vi "Lichtgitter_Referenzen_aufnehmen.vi"(8 "Fehler in":errorcluster, 11 "Cluster in":T1={"Initialisierung"={"Online?"=FALSE, "Grundpfad"=path "", "Kamera Oben"="", "IP-Adresse Flüssiglinse"="", "Flüssiglinse"=refnum, "Kamera Unten"="", "IP-Adresse SPS"="", "SPS-Verbindung"={"TCP Connection Ref"=refnum, "IP address"="", "timeout ms"=5000, "Connected?"=FALSE, "PLC Type"=enum."S7 1200", "Rack S7 400"=0, "Slot S7 400"=0, "PDU Size"=0, "connection semaphore"=refnum}, "IP-Adresse Lichtgitter"="", "Lichtgitter"=refnum, "Skalierungsfaktor"=0.0, "Bilder Oben"=[], "Bild Unten"=refnum, "Bild Ausschnitt Unten"=refnum}, "Einstellungen"={"Gesamtablauf gestartet"=FALSE, "i. O. Bilder speichern"=FALSE, "Bildspeicherung Offline"=FALSE, "Ausgewähltes Offline-Datum"="", "Ausgewähltes Offline-Teil"="", "Speicherpfad Bilder"=path ""}, "Artikeldaten"={"Artikelnummer"="", "Fertigungsauftrag"="", "Muster ISO"=refnum, "Belichtungszeit Referenzmarken"=0.0, "Fokus Referenzmarken"=0.0, "Belichtungszeit ISO"=0.0, "Fokus ISO"=0.0, "Belichtungszeit Unten"=0.0, "Kontaktanzahl"=0, "Aktueller Kontakt"=0, "Kontaktposition"={"x"=0.0, "y"=0.0}, "ISO-Muster nicht vorhanden"=FALSE, "Winkel ISO"=0.0, "Mittelpunkt ISO"={"x"=0.0, "y"=0.0}}, "Werte Kamera Oben"={"Koordinatensystem"={"Punkt x-Achse"={"X"=0.0, "Y"=0.0}, "Ursprung"={"X"=0.0, "Y"=0.0}, "Punkt y-Achse"={"X"=0.0, "Y"=0.0}}, "Position Kontakt"={"x"=0.0, "y"=0.0}, "Durchmesser Loch"=0.0, "Winkel Kontakt"=0.0, "Position Kontakt umgerechnet"={"x"=0.0, "y"=0.0}}, "Werte Kamera Unten"={"Prüfung Unten n. i. O."=FALSE}, "Werte Lichtgitter"={"Messwerte Referenzmarken"=[], "Mittelpunkt Referenzmarken"={"x"=0.0, "y"=0.0}, "Messwerte Kontakt"=[], "Offset"={"x"=0.0, "y"=0.0}}, "Rückmeldungen"={"Koordinaten ermittelt"=FALSE, "Vermessung Lichtgitter fertig"=FALSE, "Nachkontrolle Kamera Unten fertig"=FALSE}, "Fehler"={"Referenzen nicht gefunden"=FALSE, "Kontakt nicht gefunden"=FALSE, "Referenzen nicht in Lichtgitter"=FALSE, "Kontakt zu groß"=FALSE, "Kontakt zu klein"=FALSE}, "Statistik"={"Statistiken"=[]}, "Timer"={"Timer Start Position"=0, "Timer Start Lichtgitter"=0, "Timer Start Kamera Unten"=0}}) -> (0 "Fehler out":errorcluster, 3 "Cluster out":T1={"Initialisierung"={"Online?"=FALSE, "Grundpfad"=path "", "Kamera Oben"="", "IP-Adresse Flüssiglinse"="", "Flüssiglinse"=refnum, "Kamera Unten"="", "IP-Adresse SPS"="", "SPS-Verbindung"={"TCP Connection Ref"=refnum, "IP address"="", "timeout ms"=5000, "Connected?"=FALSE, "PLC Type"=enum."S7 1200", "Rack S7 400"=0, "Slot S7 400"=0, "PDU Size"=0, "connection semaphore"=refnum}, "IP-Adresse Lichtgitter"="", "Lichtgitter"=refnum, "Skalierungsfaktor"=0.0, "Bilder Oben"=[], "Bild Unten"=refnum, "Bild Ausschnitt Unten"=refnum}, "Einstellungen"={"Gesamtablauf gestartet"=FALSE, "i. O. Bilder speichern"=FALSE, "Bildspeicherung Offline"=FALSE, "Ausgewähltes Offline-Datum"="", "Ausgewähltes Offline-Teil"="", "Speicherpfad Bilder"=path ""}, "Artikeldaten"={"Artikelnummer"="", "Fertigungsauftrag"="", "Muster ISO"=refnum, "Belichtungszeit Referenzmarken"=0.0, "Fokus Referenzmarken"=0.0, "Belichtungszeit ISO"=0.0, "Fokus ISO"=0.0, "Belichtungszeit Unten"=0.0, "Kontaktanzahl"=0, "Aktueller Kontakt"=0, "Kontaktposition"={"x"=0.0, "y"=0.0}, "ISO-Muster nicht vorhanden"=FALSE, "Winkel ISO"=0.0, "Mittelpunkt ISO"={"x"=0.0, "y"=0.0}}, "Werte Kamera Oben"={"Koordinatensystem"={"Punkt x-Achse"={"X"=0.0, "Y"=0.0}, "Ursprung"={"X"=0.0, "Y"=0.0}, "Punkt y-Achse"={"X"=0.0, "Y"=0.0}}, "Position Kontakt"={"x"=0.0, "y"=0.0}, "Durchmesser Loch"=0.0, "Winkel Kontakt"=0.0, "Position Kontakt umgerechnet"={"x"=0.0, "y"=0.0}}, "Werte Kamera Unten"={"Prüfung Unten n. i. O."=FALSE}, "Werte Lichtgitter"={"Messwerte Referenzmarken"=[], "Mittelpunkt Referenzmarken"={"x"=0.0, "y"=0.0}, "Messwerte Kontakt"=[], "Offset"={"x"=0.0, "y"=0.0}}, "Rückmeldungen"={"Koordinaten ermittelt"=FALSE, "Vermessung Lichtgitter fertig"=FALSE, "Nachkontrolle Kamera Unten fertig"=FALSE}, "Fehler"={"Referenzen nicht gefunden"=FALSE, "Kontakt nicht gefunden"=FALSE, "Referenzen nicht in Lichtgitter"=FALSE, "Kontakt zu groß"=FALSE, "Kontakt zu klein"=FALSE}, "Statistik"={"Statistiken"=[]}, "Timer"={"Timer Start Position"=0, "Timer Start Lichtgitter"=0, "Timer Start Kamera Unten"=0}})   [LabVIEW 2024]
uses:
  Typdefinitionen/Cluster.ctl
  <vilib>/userDefined/High Color/IMAQdx.ctl
  <vilib>/DATA AHEAD/SP7/typedefs/S7 Connection.ctl
  <vilib>/DATA AHEAD/SP7/typedefs/PLC Type.ctl
  <vilib>/vision/Image Controls.llb/IMAQ Image.ctl
  Typdefinitionen/Koordinatensystem.ctl
  Typdefinitionen/Statistik.ctl
  <vilib>/Utility/file.llb/Read Delimited Spreadsheet (DBL).vi
  <vilib>/DATA AHEAD/SP7/SP7.lvlib
panel:
  out "Zeit":u32
  out "Anzahl Kanten":i32[](array[numeric])
  out "Lese- und Schreibestrings":string
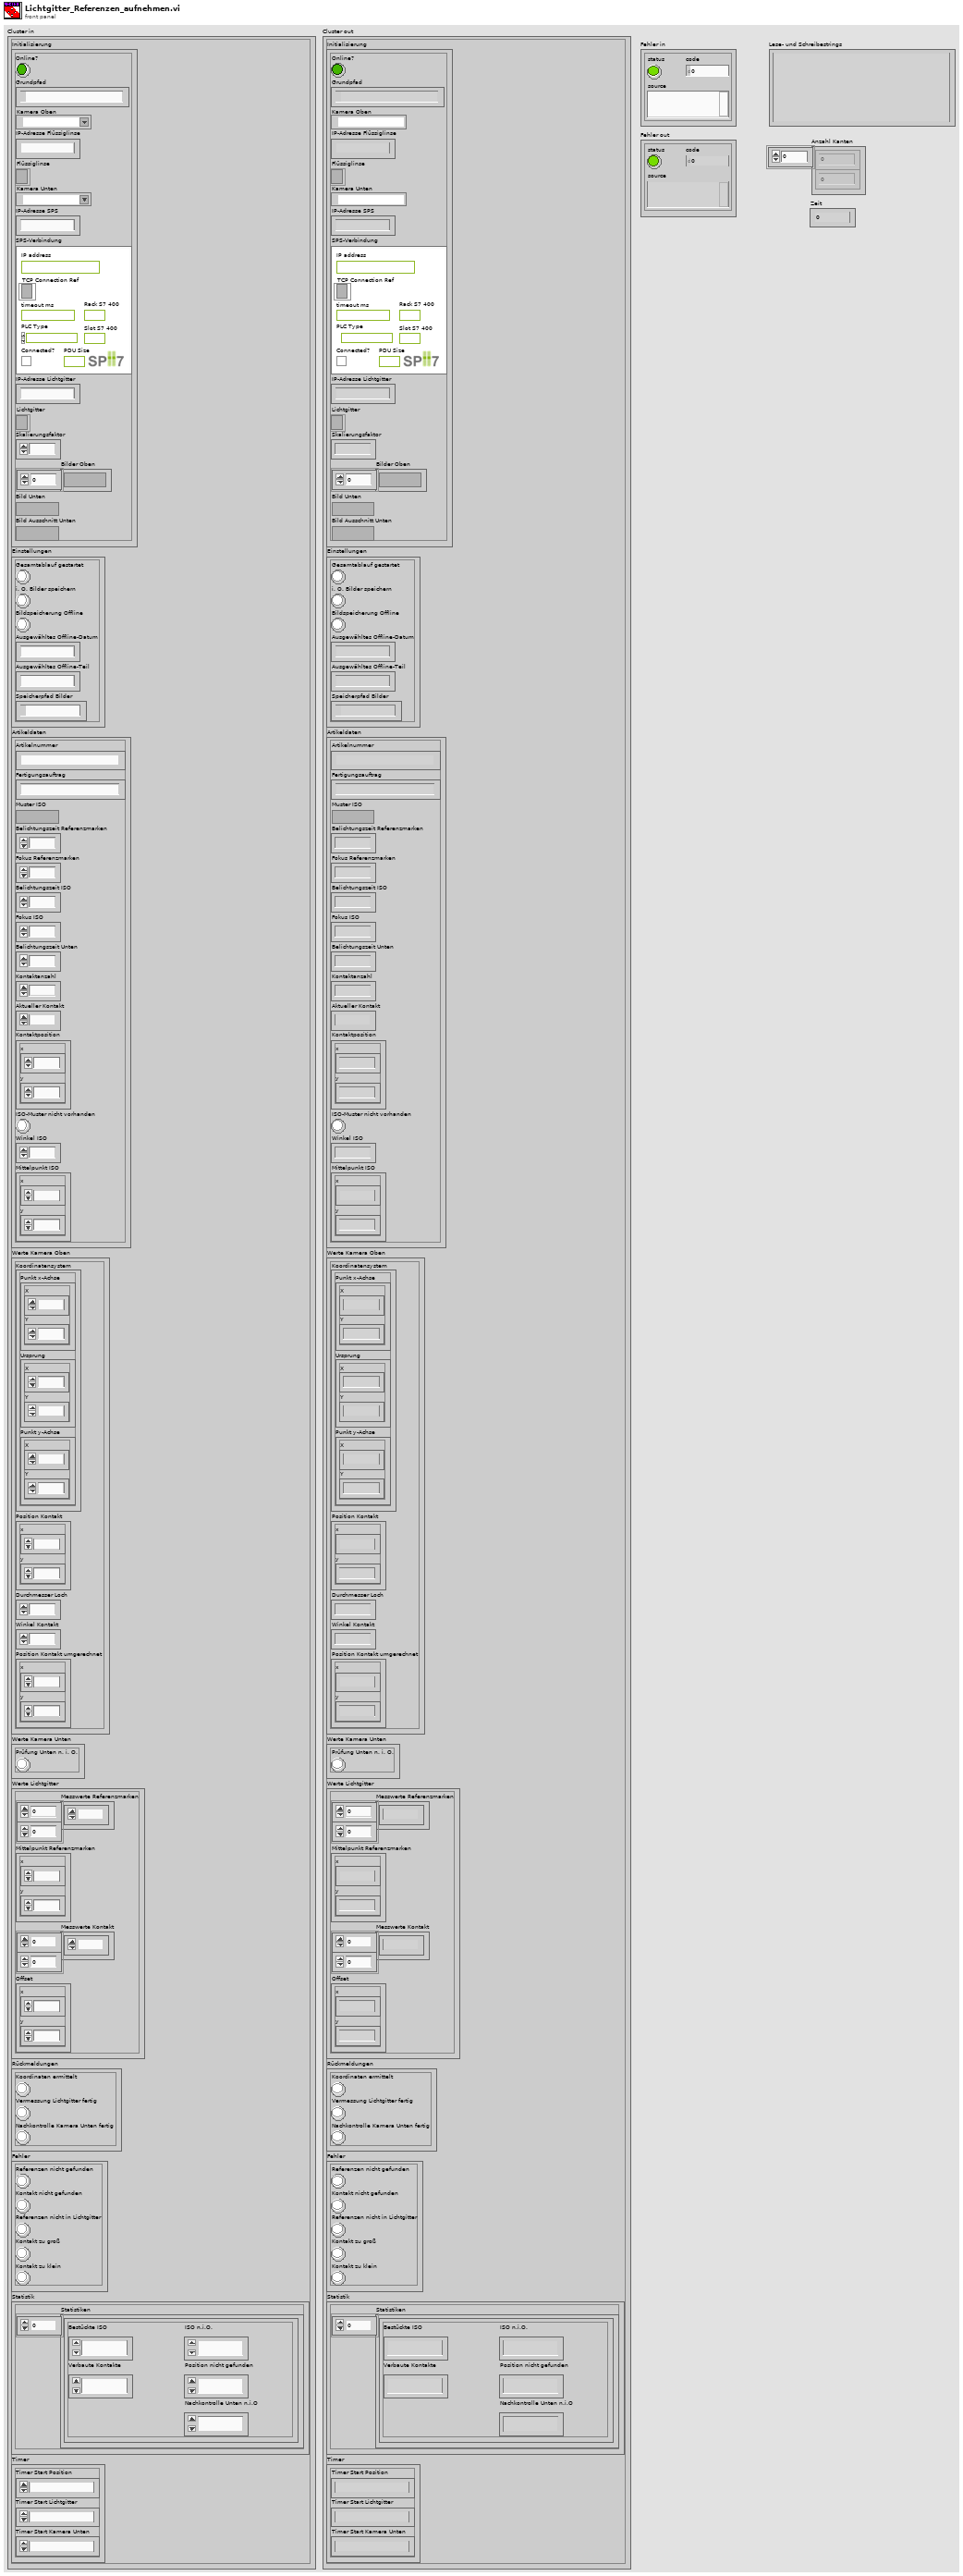
[diagram p1: front panel]
types:
  T1 = typedef "Cluster.ctl" = cluster{"Initialisierung":cluster{"Online?":bool, "Grundpfad":path, "Kamera Oben":T2, "IP-Adresse Flüssiglinse":string, "Flüssiglinse":refnum<k5>, "Kamera Unten":T2, "IP-Adresse SPS":string, "SPS-Verbindung":T3, "IP-Adresse Lichtgitter":string, "Lichtgitter":refnum<k5>, "Skalierungsfaktor":dbl, "Bilder Oben":T6[], "Bild Unten":T6, "Bild Ausschnitt Unten":T6}, "Einstellungen":cluster{"Gesamtablauf gestartet":bool, "i. O. Bilder speichern":bool, "Bildspeicherung Offline":bool, "Ausgewähltes Offline-Datum":string, "Ausgewähltes Offline-Teil":string, "Speicherpfad Bilder":path}, "Artikeldaten":cluster{"Artikelnummer":string, "Fertigungsauftrag":string, "Muster ISO":T6, "Belichtungszeit Referenzmarken":dbl, "Fokus Referenzmarken":dbl, "Belichtungszeit ISO":dbl, "Fokus ISO":dbl, "Belichtungszeit Unten":dbl, "Kontaktanzahl":u32, "Aktueller Kontakt":i16, "Kontaktposition":cluster{"x":sgl, "y":sgl}, "ISO-Muster nicht vorhanden":bool, "Winkel ISO":sgl, "Mittelpunkt ISO":cluster{"x":dbl, "y":dbl}}, "Werte Kamera Oben":cluster{"Koordinatensystem":T7, "Position Kontakt":cluster{"x":dbl, "y":dbl}, "Durchmesser Loch":dbl, "Winkel Kontakt":dbl, "Position Kontakt umgerechnet":cluster{"x":dbl, "y":dbl}}, "Werte Kamera Unten":cluster{"Prüfung Unten n. i. O.":bool}, "Werte Lichtgitter":cluster{"Messwerte Referenzmarken":dbl[][], "Mittelpunkt Referenzmarken":cluster{"x":dbl, "y":dbl}, "Messwerte Kontakt":dbl[][], "Offset":cluster{"x":dbl, "y":dbl}}, "Rückmeldungen":cluster{"Koordinaten ermittelt":bool, "Vermessung Lichtgitter fertig":bool, "Nachkontrolle Kamera Unten fertig":bool}, "Fehler":cluster{"Referenzen nicht gefunden":bool, "Kontakt nicht gefunden":bool, "Referenzen nicht in Lichtgitter":bool, "Kontakt zu groß":bool, "Kontakt zu klein":bool}, "Statistik":cluster{"Statistiken":T8[]}, "Timer":cluster{"Timer Start Position":u32, "Timer Start Lichtgitter":u32, "Timer Start Kamera Unten":u32}}
  T2 = typedef "IMAQdx.ctl" = refnum<k21>
  T3 = typedef "SP7.lvlib/S7 Connection.ctl" = cluster{"TCP Connection Ref":refnum<k5>, "IP address":string, "timeout ms":i32, "Connected?":bool, "PLC Type":T4, "Rack S7 400":u8, "Slot S7 400":u8, "PDU Size":u16, "connection semaphore":T5}
  T4 = typedef "SP7.lvlib/PLC Type.ctl" = enum16{"S7 200", "S7 300/400", "S7 1200", "S7 1500", "LOGO!8"}
  T5 = typedef "Semaphore RefNum" = refnum<k1>
  T6 = typedef "IMAQ Image.ctl" = refnum<image>
  T7 = typedef "Koordinatensystem.ctl" = cluster{"Punkt x-Achse":cluster{"X":sgl, "Y":sgl}, "Ursprung":cluster{"X":sgl, "Y":sgl}, "Punkt y-Achse":cluster{"X":sgl, "Y":sgl}}
  T8 = typedef "Statistik.ctl" = cluster{"Bestückte ISO":u32, "Verbaute Kontakte":u32, "ISO n.i.O.":u32, "Nachkontrolle Unten n.i.O":u32, "Position nicht gefunden":u32}
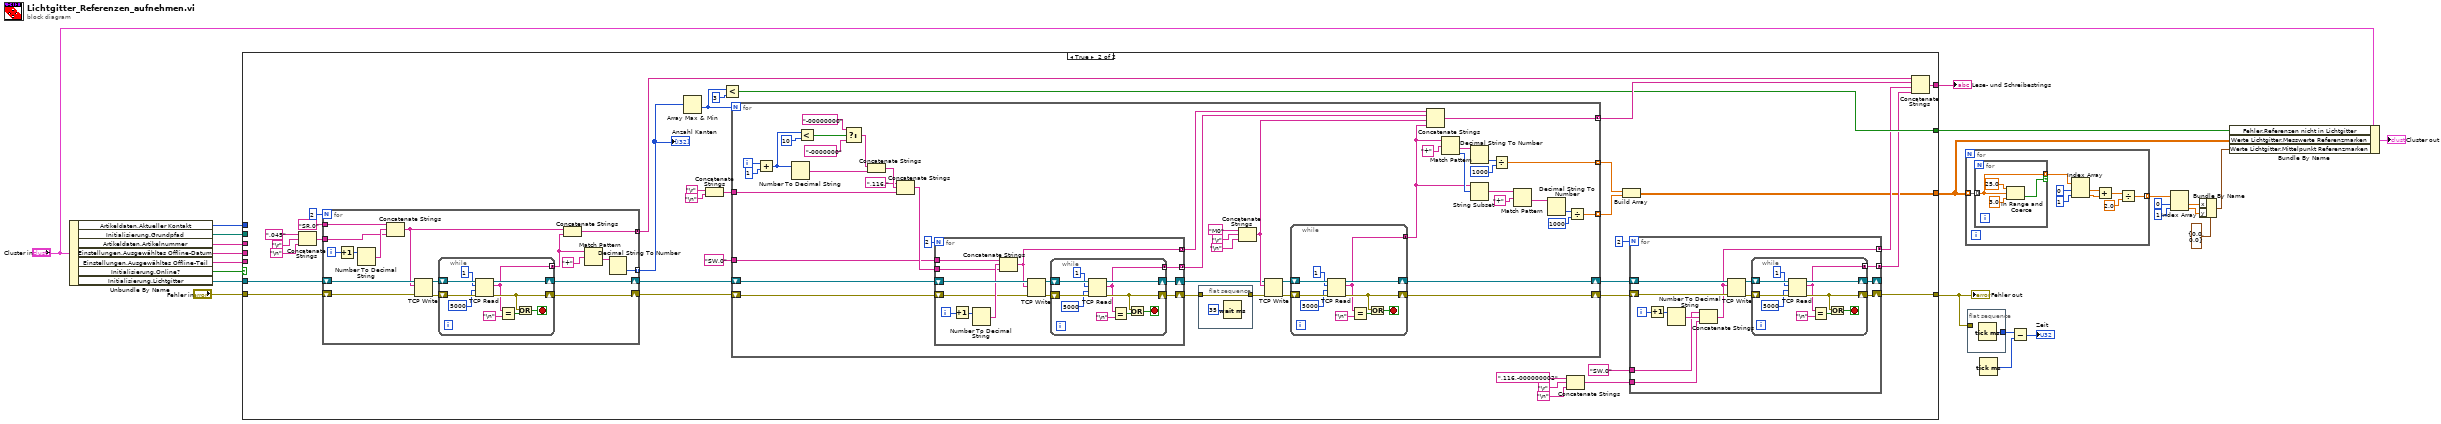
[diagram p0: block diagram]
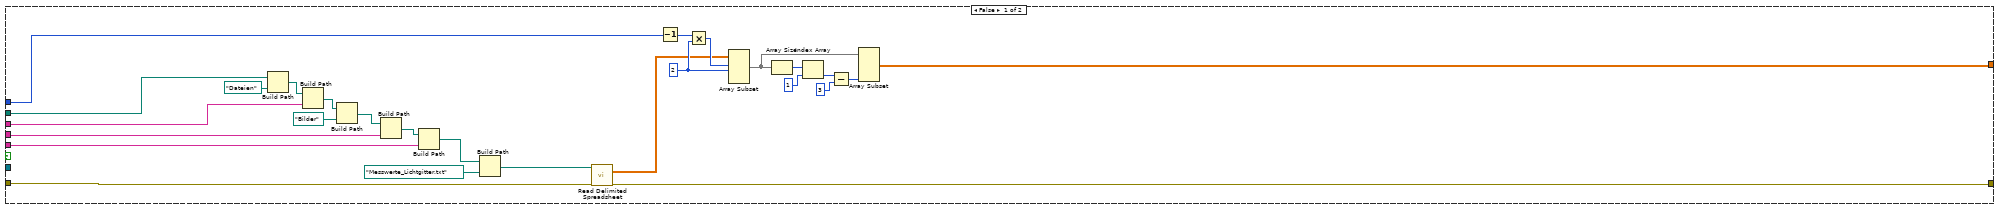
[diagram p2: hidden frame]
diagram:
  n1 = Unbundle By Name("Cluster in") -> ("Artikeldaten.Aktueller Kontakt"=w18:i16, "Initialisierung.Grundpfad"=w20:path, "Artikeldaten.Artikelnummer"=w19:string, "Einstellungen.Ausgewähltes Offline-Datum"=w21:string, "Einstellungen.Ausgewähltes Offline-Teil"=w22:string, "Initialisierung.Online?"=w23:bool, "Initialisierung.Lichtgitter"=w24:refnum<k5>)
  n2 = case shown="True" w23 {
    tunnel: [_ w73] -> w16
    tunnel: [w43 w64] -> w15
    tunnel: w24 -> [_ w69]
    tunnel: [_ w68] -> w1
    tunnel: w22 -> [w48 _]
    tunnel: w20 -> [w37 _]
    tunnel: w21 -> [w49 _]
    tunnel: w19 -> [w34 _]
    tunnel: "Fehler in" -> [w44 w67]
    tunnel: w18 -> [w42 _]
    tunnel: [w28 w52] -> w2
    frame False {
      w40 = 2 ("length")
      n3 = Build Path(base path=w37, name or relative path=path "Dateien") -> (appended path=w36:path)
      n4 = Build Path(base path=w36, name or relative path=w34) -> (appended path=w51:path)
      n5 = Build Path(base path=w51, name or relative path=path "Bilder") -> (appended path=w38:path)
      n6 = Build Path(base path=w38, name or relative path=w49) -> (appended path=w50:path)
      n7 = Build Path(base path=w50, name or relative path=w48) -> (appended path=w47:path)
      n8 = Build Path(base path=w47, name or relative path=path "Messwerte_Lichtgitter.txt") -> (appended path=w45:path)
      n9 = call-poly <vilib>:"Read Delimited Spreadsheet.vi"("file path (dialog if empty)"=w45, "error in (no error)"=w44) -> ("all rows"=w29:dbl[][], "error out"=w43:errorcluster)  [unwired: 8 in, 4 out]
      n10 = Decrement(x=w42) -> (x-1=w41:i16)
      n11 = Multiply(x=w41, y=w40) -> (x*y=w39:i32)
      n12 = Array Subset(array=w29, index (row)=w39, length (row)=w40) -> (w30:dbl[][])  [unwired: 2 in]
      n13 = Array Size(array=w30) -> (size(s)=w32:i32[])
      n14 = Index Array(array=w32, index=1) -> (element=w27:i32)
      n15 = Subtract(x=w27, y=3) -> (x-y=w26:i32)
      n16 = Array Subset(array=w30, length (col)=w26) -> (w28:dbl[][])  [unwired: 3 in]
    }
    frame True {
      n17 = Concatenate Strings(",045" ("string"), "\r", "\n") -> (w82:string)
      n18 = for {
        N: 2 -> [_]
        tunnel: "SR,0" ("string") -> [w198]
        shift-right: [w201] -> w77
        shift-left: w69 -> [w199]
        shift-right: [w200] -> w81
        shift-left: w67 -> [w195]
        tunnel: w82 -> [w196]
        tunnel: [w193] -> w74 mode=concatenating
        tunnel: [w189] -> w53 mode=indexing
        i -> [w203]
        n19 = Increment(x=w203) -> (x+1=w202:i32)
        n20 = Number To Decimal String(number=w202) -> (decimal integer string=w197:string)  [unwired: 1 in]
        n21 = Concatenate Strings(w198, w197, w196) -> (w194:string)
        n22 = TCP Write(connection ID=w199, data in=w194, error in (no error)=w195) -> (connection ID out=w204:refnum<k5>, error out=w205:errorcluster)  [unwired: 1 in, 1 out]
        n23 = while {
          shift-right: [w213] -> w201
          shift-left: w204 -> [w215]
          shift-right: [w209] -> w200
          shift-left: w205 -> [w214]
          tunnel: [w206] -> w190 mode=concatenating
          stop <- w208 stop-if-true
          n24 = TCP Read(connection ID=w215, bytes to read=1, error in (no error)=w214, 9:5000 ("timeout ms (25000)")) -> (connection ID out=w213:refnum<k5>, data out=w206:string, error out=w209:errorcluster)  [unwired: 1 in]
          n25 = Equal?(x=w206, y="\n") -> (x = y?=w210:bool)
          n26 = Or(x=w209, y=w210) -> (x .or. y?=w208:bool)
        }
        n27 = Concatenate Strings(w194, w190) -> (w193:string)
        n28 = Match Pattern(string=w190, regular expression="+" ("search string")) -> (after substring=w192:string)  [unwired: 1 in, 3 out]
        n29 = Decimal String To Number(string=w192) -> (number=w189:i32)  [unwired: 2 in, 1 out]
      }
      "Anzahl Kanten" <- w53
      n30 = Array Max & Min(array=w53) -> (min value=w55:i32)  [unwired: 3 out]
      n31 = Concatenate Strings("\r", "\n") -> (w78:string)
      n32 = Less?(x=w55, y=3 ("x")) -> (x < y?=w68:bool)
      n33 = for {
        N: w55 -> [_]
        shift-right: [w114] -> w66
        shift-left: w77 -> [w110]
        shift-right: [w115] -> w65
        shift-left: w81 -> [w117]
        tunnel: w78 -> [w153]
        tunnel: [w149] -> w75 mode=concatenating
        tunnel: [w129] -> w70 mode=indexing
        tunnel: "SW,0" ("string") -> [w125]
        tunnel: [w128] -> w71 mode=indexing
        i -> [w122]
        n34 = Add(x=w122, y=1) -> (x+y=w121:i32)
        n35 = Number To Decimal String(number=w121) -> (decimal integer string=w152:string)  [unwired: 1 in]
        n36 = Less?(x=w121, y=10) -> (x < y?=w147:bool)
        n37 = Select(t="-00000000" ("string"), s=w147, f="-0000000" ("string")) -> (s? t:f=w144:string)
        n38 = Concatenate Strings(w144, w152) -> (w151:string)
        n39 = Concatenate Strings(",116," ("string"), w151, w153) -> (w126:string)
        n40 = for {
          N: 2 -> [_]
          tunnel: w125 -> [w161]
          shift-right: [w164] -> w113
          shift-left: w110 -> [w162]
          shift-right: [w163] -> w112
          shift-left: w117 -> [w158]
          tunnel: w126 -> [w159]
          tunnel: [w157] -> w124 mode=concatenating
          tunnel: [w156] -> w123 mode=concatenating
          i -> [w166]
          n41 = Increment(x=w166) -> (x+1=w165:i32)
          n42 = Number To Decimal String(number=w165) -> (decimal integer string=w160:string)  [unwired: 1 in]
          n43 = Concatenate Strings(w161, w160, w159) -> (w156:string)
          n44 = TCP Write(connection ID=w162, data in=w156, error in (no error)=w158) -> (connection ID out=w167:refnum<k5>, error out=w168:errorcluster)  [unwired: 1 in, 1 out]
          n45 = while {
            shift-right: [w176] -> w164
            shift-left: w167 -> [w178]
            shift-right: [w172] -> w163
            shift-left: w168 -> [w177]
            tunnel: [w169] -> w157 mode=concatenating
            stop <- w171 stop-if-true
            n46 = TCP Read(connection ID=w178, bytes to read=1, error in (no error)=w177, 9:5000 ("timeout ms (25000)")) -> (connection ID out=w176:refnum<k5>, data out=w169:string, error out=w172:errorcluster)  [unwired: 1 in]
            n47 = Equal?(x=w169, y="\n") -> (x = y?=w173:bool)
            n48 = Or(x=w172, y=w173) -> (x .or. y?=w171:bool)
          }
        }
        n49 = flat-sequence {
          tunnel: w112 -> [w155]
          tunnel: [w155] -> w111
          frame #0 {
            n50 = Wait (ms)(milliseconds to wait=u32 35) -> ()  [unwired: 1 out]
          }
        }
        n51 = Concatenate Strings("M0" ("string"), "\r", "\n") -> (w116:string)
        n52 = TCP Write(connection ID=w113, data in=w116, error in (no error)=w111) -> (connection ID out=w139:refnum<k5>, error out=w140:errorcluster)  [unwired: 1 in, 1 out]
        n53 = while {
          shift-right: [w186] -> w114
          shift-left: w139 -> [w188]
          shift-right: [w182] -> w115
          shift-left: w140 -> [w187]
          tunnel: [w179] -> w119 mode=concatenating
          stop <- w181 stop-if-true
          n54 = TCP Read(connection ID=w188, bytes to read=1, error in (no error)=w187, 9:5000 ("timeout ms (25000)")) -> (connection ID out=w186:refnum<k5>, data out=w179:string, error out=w182:errorcluster)  [unwired: 1 in]
          n55 = Equal?(x=w179, y="\n") -> (x = y?=w183:bool)
          n56 = Or(x=w182, y=w183) -> (x .or. y?=w181:bool)
        }
        n57 = Concatenate Strings(w123, w124, w116, w119) -> (w149:string)
        n58 = Match Pattern(string=w119, regular expression="+") -> (after substring=w137:string, offset past match=w127:i32)  [unwired: 1 in, 2 out]
        n59 = Decimal String To Number(string=w137) -> (number=w138:i32)  [unwired: 2 in, 1 out]
        n60 = String Subset(string=w119, offset (0)=w127) -> (substring=w134:string)  [unwired: 1 in]
        n61 = Divide(x=w138, y=1000) -> (x/y=w128:dbl)
        n62 = Match Pattern(string=w134, regular expression="+") -> (after substring=w130:string)  [unwired: 1 in, 3 out]
        n63 = Decimal String To Number(string=w130) -> (number=w131:i32)  [unwired: 2 in, 1 out]
        n64 = Divide(x=w131, y=1000) -> (x/y=w129:dbl)
      }
      n65 = Concatenate Strings(",116,-000000002" ("string"), "\r", "\n") -> (w59:string)
      n66 = Build Array(w71, w70) -> (w52:dbl[][])
      n67 = for {
        N: 2 -> [_]
        shift-right: [w95] -> _
        shift-left: w66 -> [w93]
        shift-right: [w94] -> w64
        shift-left: w65 -> [w91]
        tunnel: [w90] -> w57 mode=concatenating
        tunnel: [w89] -> w58 mode=concatenating
        tunnel: "SW,0" ("string") -> [w88]
        tunnel: w59 -> [w87]
        i -> [w97]
        n68 = Increment(x=w97) -> (x+1=w96:i32)
        n69 = Number To Decimal String(number=w96) -> (decimal integer string=w92:string)  [unwired: 1 in]
        n70 = Concatenate Strings(w88, w92, w87) -> (w89:string)
        n71 = TCP Write(connection ID=w93, data in=w89, error in (no error)=w91) -> (connection ID out=w98:refnum<k5>, error out=w99:errorcluster)  [unwired: 1 in, 1 out]
        n72 = while {
          shift-right: [w107] -> w95
          shift-left: w98 -> [w109]
          shift-right: [w103] -> w94
          shift-left: w99 -> [w108]
          tunnel: [w100] -> w90 mode=concatenating
          stop <- w102 stop-if-true
          n73 = TCP Read(connection ID=w109, bytes to read=1, error in (no error)=w108, 9:5000 ("timeout ms (25000)")) -> (connection ID out=w107:refnum<k5>, data out=w100:string, error out=w103:errorcluster)  [unwired: 1 in]
          n74 = Equal?(x=w100, y="\n") -> (x = y?=w104:bool)
          n75 = Or(x=w103, y=w104) -> (x .or. y?=w102:bool)
        }
      }
      n76 = Concatenate Strings(w74, w75, w58, w57) -> (w73:string)
    }
  }
  "Fehler out" <- w15
  "Lese- und Schreibestrings" <- w16
  n77 = for {
    tunnel: w2 -> [w224] mode=indexing
    tunnel: [w216] -> w3 mode=indexing
    n78 = for {
      tunnel: w224 -> [w226] mode=indexing
      tunnel: [w226] -> w223 mode=indexing if=w225
      n79 = In Range and Coerce(upper limit=25.0, x=w226, lower limit=3.0) -> (In Range?=w225:bool)  [unwired: 1 out]
    }
    n80 = Index Array(array=w223, index #1=0 ("index"), index #2=1 ("index")) -> (element #1=w220:dbl, element #2=w219:dbl)
    n81 = Add(x=w220, y=w219) -> (x+y=w218:dbl)
    n82 = Divide(x=w218, y=2.0) -> (x/y=w216:dbl)
  }
  n83 = flat-sequence {
    tunnel: w15 -> [_]
    tunnel: [w229] -> w14
    frame #0 {
      n84 = Tick Count (ms)() -> (millisecond timer value=w229:u32)
    }
  }
  n85 = Tick Count (ms)() -> (millisecond timer value=w13:u32)
  n86 = Subtract(x=w14, y=w13) -> (x-y=→"Zeit":u32)
  n87 = Index Array(array=w3, index #1=0 ("index"), index #2=1 ("index")) -> (element #1=w8:dbl, element #2=w9:dbl)
  n88 = Bundle By Name(cluster=cluster{"x":dbl, "y":dbl} {"x"=0.0, "y"=0.0} ("Werte Lichtgitter.Mittelpunkt"), "x"=w8, "y"=w9) -> (w4:cluster{"x":dbl, "y":dbl})
  n89 = Bundle By Name(cluster="Cluster in", "Fehler.Referenzen nicht in Lichtgitter"=w1, "Werte Lichtgitter.Messwerte Referenzmarken"=w2, "Werte Lichtgitter.Mittelpunkt Referenzmarken"=w4) -> (→"Cluster out":T1)
